vi "Set Position Setpoint.vi"(8 "error in (no error)":errorcluster, 10 "position (m)":dbl, 11 "simulated KUKA youBot gripper motor in":refnum<class "NI_Robotics_KUKA youBot Gripper Motor_Sim.lvclass">) -> (0 "error out":errorcluster, 3 "simulated KUKA youBot gripper motor out":refnum<class "NI_Robotics_KUKA youBot Gripper Motor_Sim.lvclass">)   [LabVIEW 2017, in "NI_Robotics_KUKA youBot Host.lvlib" / "NI_Robotics_KUKA youBot Gripper Motor_Sim.lvclass"]
uses:
  <vilib>/robotics/KUKA youBot/Motor/Gripper Motor Sim/NI_Robotics_KUKA youBot Gripper Motor_Sim.lvclass
  c:/Program Files (x86)/National Instruments/LabVIEW 2017/vi.lib/robotics/KUKA youBot/Motor/Gripper Motor/NI_Robotics_KUKA youBot Gripper Motor.lvclass
  <vilib>/robotics/KUKA youBot/Motor/Gripper Motor Sim/NI_Robotics_KUKA youBot Gripper Motor_Sim.lvclass/NI_Robotics_KUKA youBot Gripper Motor_Sim.ctl
  <vilib>/robotics/Simulator/Robot Factory/Motor/ODESimulator_Motor.lvclass
  <vilib>/robotics/KUKA youBot/Motor/Gripper Motor/NI_Robotics_KUKA youBot Gripper Motor.lvclass
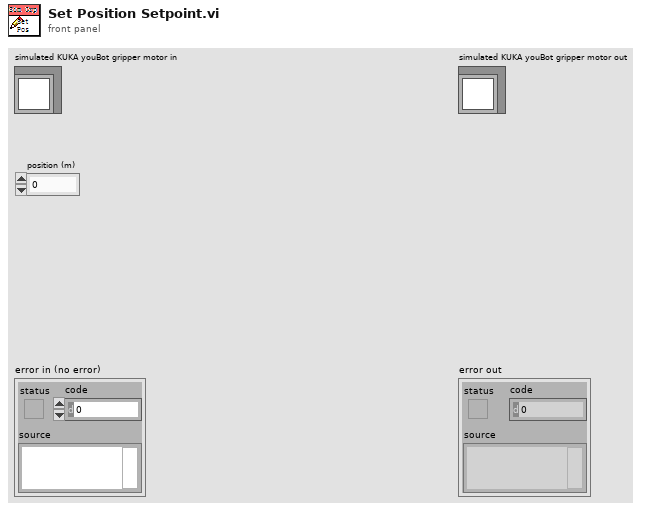
[diagram p1: front panel]
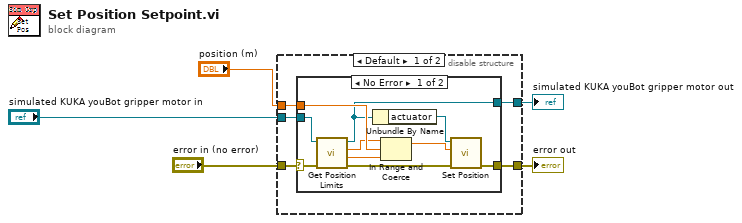
[diagram p0: block diagram]
diagram:
  n1 = disable-structure shown="Default" {
    disable-tunnel: "error in (no error)" -> [w10 w23]
    disable-tunnel: "position (m)" -> [w9 _]
    disable-tunnel: "simulated KUKA youBot gripper motor in" -> [w8 w24]
    disable-tunnel: [w7 w23] -> w1
    disable-tunnel: [w6 w24] -> w2
    frame condition #0 (active) {
      n2 = case shown="No Error" w10 {
        selector: w10 -> [w15 w21]
        tunnel: w9 -> [w20 _]
        tunnel: w8 -> [w16 w22]
        tunnel: [w19 w21] -> w7
        tunnel: [w11 w22] -> w6
        frame No Error {
          n3 = call <vilib>:"Get Position Limits.vi"("error in (no error)"=w15, "KUKA youBot gripper motor in"=w16) -> ("error out"=w14:errorcluster, "min dist (m)"=w13:dbl, "max dist (m)"=w12:dbl, "KUKA youBot gripper motor out"=w11:refnum<class "NI_Robotics_KUKA youBot Gripper Motor_Sim.lvclass">)  [unwired: 6 in]
          n4 = Unbundle By Name(w11) -> ("actuator"=w17:refnum<class "ODESimulator_Motor.lvclass">)
          n5 = In Range and Coerce(upper limit=w12, x=w20, lower limit=w13) -> (coerced(x)=w18:dbl)  [unwired: 1 out]
          n6 = call-dynamic "Set Position.vi"("error in (no error)"=w14, "CCW Position (0.0 rad)"=w18, "Motor in"=w17) -> ("error out"=w19:errorcluster)  [unwired: 7 in, 1 out]
        }
        frame Error {
        }
      }
    }
    frame condition #1 {
    }
  }
  "error out" <- w1
  "simulated KUKA youBot gripper motor out" <- w2
